vi "Internal Init.vi"(4 "reset device (boolean value)":bool, 5 "topology suffix (none)":string, 6 "device":refnum<k21>, 7 "Topology":string, 8 "error in (no error)":errorcluster, 9 "NVMEM Session":refnum<class "SLSC Interface.lvclass">, 10 "No Resource Session":refnum<class "SLSC Interface.lvclass">, 11 "SLSC Switch in":refnum<class "SLSC Switch.lvclass">) -> (0 "error out":errorcluster, 3 "SLSC Switch out":refnum<class "SLSC Switch.lvclass">)   [LabVIEW 2017, in "SLSC Switch.lvlib" / "SLSC Switch.lvclass"]
uses:
  SLSC Switch.lvclass
  <vilib>/National Instruments/SLSC Local or Remote Interface/SLSC Interface Class/SLSC Interface.lvclass
  SLSC Switch.lvclass/SLSC Switch.ctl
  <vilib>/Utility/error.llb/Clear Errors.vi
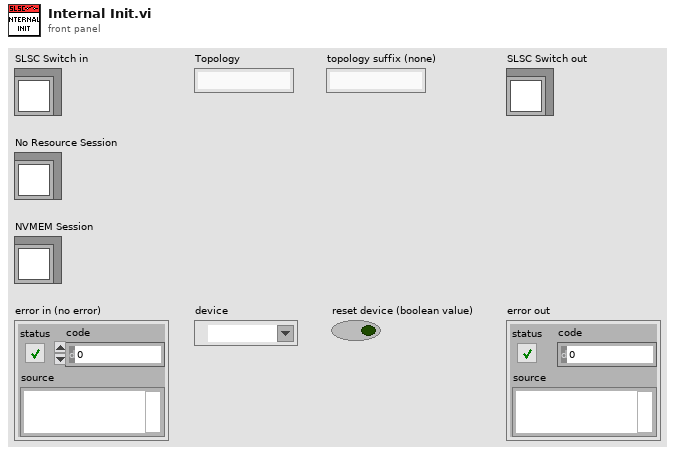
[diagram p1: front panel]
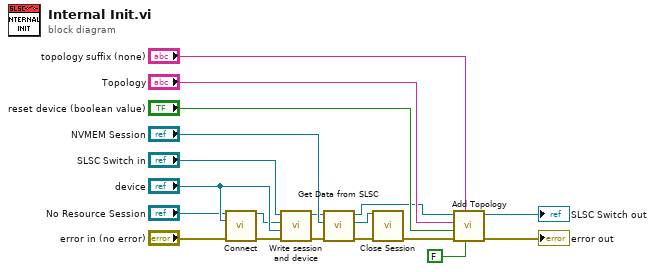
[diagram p0: block diagram]
diagram:
  n1 = call-dynamic "Connect.vi"("SLSC Interface in"="No Resource Session", "devices"="device", "error in (no error)"="error in (no error)") -> ("SLSC Interface out"=w13:refnum<class "SLSC Interface.lvclass">, "error out"=w9:errorcluster)  [unwired: 11 in]
  n2 = call "Write session and device.vi"("error in (no error)"=w9, "SLSC Device"="device", "SLSC Session in"=w13, "SLSC Switch in"="SLSC Switch in") -> ("error out"=w2:errorcluster, "SLSC Switch out"=w3:refnum<class "SLSC Switch.lvclass">)  [unwired: 6 in]
  n3 = call "Get Data from SLSC.vi"("error in (no error)"=w2, "SLSC NVMEM Session In"="NVMEM Session", "SLSC Switch in"=w3) -> ("error out"=w17:errorcluster, "SLSC NVMEM Session Out"=w16:refnum<class "SLSC Interface.lvclass">, "SLSC Switch out"=w4:refnum<class "SLSC Switch.lvclass">)  [unwired: 6 in]
  n4 = call-dynamic "Close Session.vi"("SLSC Interface in"=w16, "error in (no error)"=w17) -> ("error out"=w18:errorcluster)  [unwired: 13 in]
  n5 = call "Add Topology.vi"("Append to Active?"=FALSE, "topology suffix (none)"="topology suffix (none)", "error in (no error)"=w18, "reset device (boolean value)"="reset device (boolean value)", "Topology"="Topology", "SLSC Switch in"=w4) -> ("error out"=→"error out":errorcluster, "SLSC Switch out"=→"SLSC Switch out":refnum<class "SLSC Switch.lvclass">)  [unwired: 4 in]
